vi "ShoulderExecute.vi"(8 "error in (no error)":errorcluster) -> (0 "error out":errorcluster)   [LabVIEW 2023]
doc: "Arm Execute for 2024 robot"
uses:
  <vilib>/Rock Robotics/WPI/ThirdParty/JAS_Junk/TrajLib/Trajectory_Library.lvlib
  ShoulderGetSetpointEnum.ctl
  Unused_OldRobot/ShoulderNetworkingGlobal.vi
  ShoulderGlobal.vi
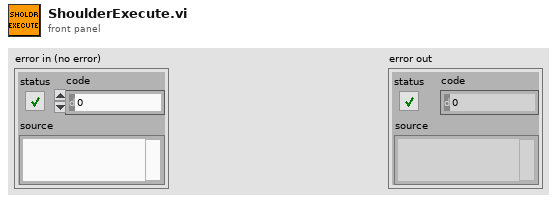
[diagram p1: front panel]
types:
  T1 = typedef "WPI_MotorControlDeviceRef.ctl" = cluster{"DeviceStatus":errorcluster, "Type":T2, "PWM":cluster{"PWM Channel":T3, "DeadBand":T4}, "CAN":cluster{"Device Number":u8, "SetOutput VI Ref":variant, "GetOutput VI Ref":variant, "Enable VI Ref":variant, "Disable VI Ref":variant, "Data":variant}, "Invert":bool, "DIO PWM":cluster{"PWM \"Enable\" Channel":T3, "DIOChannel":T5, "PWM Rate":dbl}}
  T2 = typedef "WPI_MotorControlType.ctl" = enum16{"PWM", "CAN", "DIO PWM"}
  T3 = typedef "FPGA_DIOPWMChannel.ctl" = enum8{"PWM 0", "PWM 1", "PWM 2", "PWM 3", "PWM 4", "PWM 5", "PWM 6", "PWM 7", "PWM 8", "PWM 9", "PWM MXP 0", "PWM MXP 1", "PWM MXP 2", "PWM MXP 3", "PWM MXP 4", "PWM MXP 5", "PWM MXP 6", "PWM MXP 7", "PWM MXP 8", "PWM MXP 9", "Invalid"}
  T4 = typedef "WPI_PWMDeadband.ctl" = cluster{"Name":string, "maxPositivePwm":i32, "minPositivePwm":i32, "centerPwm":i32, "maxNegativePwm":i32, "minNegativePwm":i32, "angularRange":u16}
  T5 = typedef "FPGA_DIOChannel.ctl" = enum8{"DIO 0", "DIO 1", "DIO 2", "DIO 3", "DIO 4", "DIO 5", "DIO 6", "DIO 7", "DIO 8", "DIO 9", "DIO MXP 0", "DIO MXP 1", "DIO MXP 2", "DIO MXP 3", "DIO MXP 4", "DIO MXP 5", "DIO MXP 6", "DIO MXP 7", "DIO MXP 8", "DIO MXP 9", "DIO MXP 10", "DIO MXP 11", "DIO MXP 12", "DIO MXP 13", "DIO MXP 14", "DIO MXP 15", "SPI Port CS1", "SPI Port CS2", "SPI Port CS3", "SPI Port MISO", "SPI Port MOSI", "Invalid"}
  T6 = typedef "WPI_SwitchDevRef.ctl" = cluster{"DevStatus":errorcluster, "DIO Channel":T5, "CntIndex":T7, "Normally Closed":bool}
  T7 = typedef "FPGA_CounterCtrSystemIndex.ctl" = enum8{"Ctr 0", "Ctr 1", "Ctr 2", "Ctr 3", "Ctr 4", "Ctr 5", "Ctr 6", "Ctr 7", "Invalid"}
  T8 = typedef "ShoulderGetSetpointEnum.ctl" = enum16{"ShoulderRest", "ShoulderSpeaker", "ShoulderAmp"}
  T9 = typedef "Trajectory_Library.lvlib/PosCtrl_Tuning_Type.ctl" = cluster{"Slope":dbl, "Offset":dbl, "Error Deadband":dbl, "At Reference Count":i32, "Negate Output":bool, "Max Allowd Position":dbl, "Min Allowd Position":dbl}
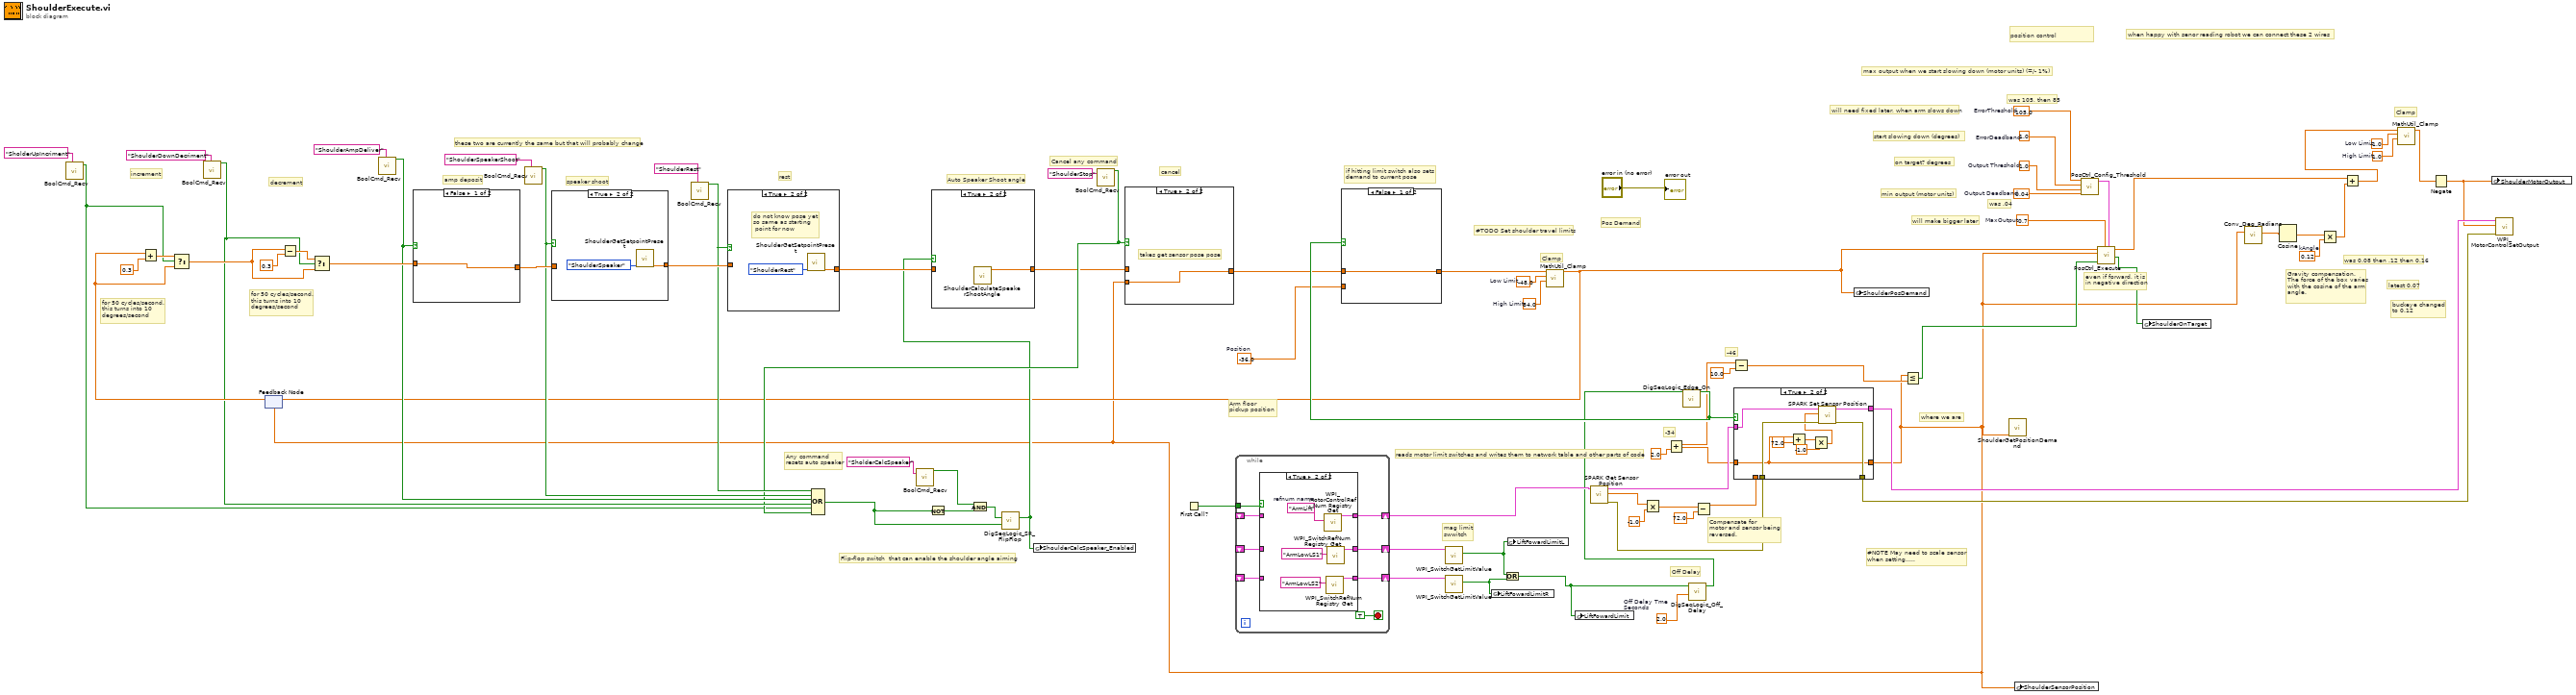
[diagram p0: block diagram]
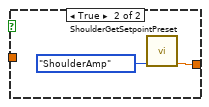
[diagram p8: hidden frame]
diagram:
  w28 = 84.0  # High Limit
  w33 = 2.0  # Off Delay Tme Seconds
  w43 = 1.0  # High Limit
  w42 = -1.0  # Low Limit
  w36 = -36.0  # Position
  w61 = 0.12  # kAngle
  w72 = -48.0  # Low Limit
  w79 = 0.7  # MaxOutput
  w77 = 105.0  # ErrorThreshold
  w76 = 1.0  # ErrorDeadband
  w75 = 1.0  # Output Threshold
  w74 = 0.04  # Output Deadband
  # "#TODO Set shoulder travel limits"
  # "Auto Speaker Shoot angle"
  # "Any command\nresets auto speaker"
  # "for 50 cycles/second.\nthis turns into 10 \ndegrees/second"
  # "for 50 cycles/second.\nthis turns into 10 \ndegrees/second"
  # "increment"
  # "buckeye changed\nto 0.12"
  # "latest 0.07"
  # "Flip-flop switch  that can enable the shoulder angle aiming"
  # "#NOTE May need to scale sensor \nwhen setting....."
  # "Off Delay"
  # "mag limit\nswwitch"
  # "-34"
  # "-46"
  # "Pos Demand"
  # "Clamp"
  # "was 105, then 85"
  # "was .04"
  # "was 0.08 then .12 then 0.16"
  # "Arm floor\npickup position"
  # "Gravity compensation.\nThe force of the box varies\nwith the cosine of the arm\nangle."
  # "Compensate for\nmotor and sensor being\nreversed."
  # "even if forward, it is \nin negative direction"
  # "if hitting limit switch also sets \ndemand to current pose"
  # "these two are currently the same but that will probably change"
  # "Cancel any command"
  # "cancel"
  # "rest"
  # "speaker shoot"
  # "Clamp"
  # "amp deposit"
  # "decrement"
  # "when happy with senor reading robot we can connect these 2 wires"
  # "min output (motor units)"
  # "max output when we start slowing down (motor units) (=/- 1%)"
  # "on target? degrees"
  # "start slowing down (degrees)"
  # "will make bigger later"
  # "where we are"
  # "position control"
  # "will need fixed later, when arm slows down"
  # "reads motor limit switches and writes them to network table and other parts of code"
  n1 = call <vilib>:"BoolCmd_Recv.vi"("Command Name"="SholderUpIncriment") -> ("New Request"=w9:bool)  [unwired: 9 in, 1 out]
  n2 = call <vilib>:"BoolCmd_Recv.vi"("Command Name"="ShoulderDownDecriment") -> ("New Request"=w11:bool)  [unwired: 9 in, 1 out]
  n3 = call <vilib>:"BoolCmd_Recv.vi"("Command Name"="ShoulderAmpDeliver") -> ("New Request"=w12:bool)  [unwired: 9 in, 1 out]
  n4 = call <vilib>:"BoolCmd_Recv.vi"("Command Name"="ShoulderSpeakerShoot") -> ("New Request"=w13:bool)  [unwired: 9 in, 1 out]
  n5 = call <vilib>:"BoolCmd_Recv.vi"("Command Name"="ShoulderRest") -> ("New Request"=w14:bool)  [unwired: 9 in, 1 out]
  n6 = call <vilib>:"BoolCmd_Recv.vi"("Command Name"="SholderCalcSpeaker") -> ("New Request"=w15:bool)  [unwired: 9 in, 1 out]
  n7 = call <vilib>:"BoolCmd_Recv.vi"("Command Name"="ShoulderStop") -> ("New Request"=w10:bool)  [unwired: 9 in, 1 out]
  n8 = Compound Arithmetic op=OR(w14, w13, w12, w11, w9, w10) -> (w8:bool)
  n9 = Not(x=w8) -> (.not. x?=w30:bool)
  n10 = And(x=w15, y=w30) -> (x .and. y?=w29:bool)
  n11 = call <vilib>:"DigSeqLogic_SR_FlipFlop.vi"("Set"=w29, "Reset"=w8) -> ("Output"=w6:bool)  [unwired: 12 in, 1 out]
  n12 = global write "ShoulderGlobal.vi" "ShoulderCalcSpeaker_Enabled"(w6) -> ()
  n13 = First Call?() -> (First Call?: T/F=w49:bool)
  n14 = while {
    tunnel: w49 -> [w86]
    shift-right: [w87] -> w44
    shift-left: _ -> [w84]
    shift-right: [w83] -> w47
    shift-left: _ -> [w82]
    shift-right: [w81] -> w27
    shift-left: _ -> [w80]
    stop <- TRUE stop-if-true
    n15 = case shown="True" w86 {
      tunnel: [w90 w96] -> w87
      tunnel: w84 -> [w90 _]
      tunnel: [w89 w93] -> w83
      tunnel: w82 -> [w89 _]
      tunnel: [w88 w91] -> w81
      tunnel: w80 -> [w88 _]
      frame False {
      }
      frame True {
        w95 = "ArmLift"  # refnum name
        n16 = call <vilib>:"WPI_MotorControlRefNum Registry Get.vi"("refnum name"=w95) -> ("MotorControlDevRef"=w96:T1)  [unwired: 9 in, 1 out]
        n17 = call <vilib>:"WPI_SwitchRefNum Registry Get.vi"("refnum name"="ArmLowLS2") -> ("SwitchDevRef"=w91:T6)  [unwired: 9 in, 1 out]
        n18 = call <vilib>:"WPI_SwitchRefNum Registry Get.vi"("refnum name"="ArmLowLS1") -> ("SwitchDevRef"=w93:T6)  [unwired: 9 in, 1 out]
      }
    }
  }
  n19 = call <vilib>:"WPI_SwitchGetLimitValue.vi"("SwitchDevRef"=w47) -> ("Switch Pressed"=w26:bool)  [unwired: 8 in, 2 out]
  n20 = call <vilib>:"WPI_SwitchGetLimitValue.vi"("SwitchDevRef"=w27) -> ("Switch Pressed"=w25:bool)  [unwired: 8 in, 2 out]
  n21 = global write "ShoulderNetworkingGlobal.vi" "LiftFowardLimitR"(w25) -> ()
  n22 = Or(x=w26, y=w25) -> (x .or. y?=w24:bool)
  n23 = global write "ShoulderNetworkingGlobal.vi" "LiftFowardLimitL"(w26) -> ()
  n24 = global write "ShoulderNetworkingGlobal.vi" "LiftFowardLimit"(w24) -> ()
  n25 = call <vilib>:"SPARK Get Sensor Position.vi"("MotorControlDevRef in"=w44) -> ("error out"=w48:errorcluster, "Sensor Position"=w57:dbl, "MotorControlDevRef out"=w58:T1)  [unwired: 7 in, 1 out]
  n26 = Multiply(x=w57, y=-1.0) -> (x*y=w55:dbl)
  n27 = Add(y=2.0) -> (x=w1:dbl, x+y=w39:dbl)
  n28 = call <vilib>:"DigSeqLogic_Off_Delay.vi"("Delay"=w33, "Input"=w24) -> ("Output"=w32:bool)  [unwired: 8 in, 1 out]
  n29 = call <vilib>:"DigSeqLogic_Edge_On.vi"("Input"=w32) -> ("On Edge"=w52:bool)  [unwired: 10 in]
  n30 = Subtract(x=w55, y=72.0) -> (x-y=w53:dbl)
  n31 = Subtract(x=w1, y=10.0) -> (x-y=w34:dbl)
  n32 = call "ShoulderGetPositionDemand.vi"() -> ("ShoulderPosDmd"=w2:dbl)  [unwired: 11 in]
  n33 = feedback #1(w2) -> (w73:dbl)
  n34 = Add(x=w73, y=0.3) -> (x+y=w20:dbl)
  n35 = Select(t=w20, s=w9, f=w73) -> (s? t:f=w19:dbl)
  n36 = Subtract(x=w19, y=0.3) -> (x-y=w17:dbl)
  n37 = Select(t=w17, s=w11, f=w19) -> (s? t:f=w23:dbl)
  n38 = case shown="False" w12 {
    tunnel: w23 -> [w97 _]
    tunnel: [w97 w98] -> w71
    frame False {
    }
    frame True {
      n39 = call "ShoulderGetSetpointPreset.vi"("SholdrSetpoints"=ShoulderGetSetpointEnum."ShoulderAmp" ("ArmSetpoints")) -> ("Setpoint"=w98:dbl)  [unwired: 10 in]
    }
  }
  n40 = case shown="True" w13 {
    tunnel: w71 -> [w100 _]
    tunnel: [w100 w102] -> w22
    frame False {
    }
    frame True {
      n41 = call "ShoulderGetSetpointPreset.vi"("SholdrSetpoints"=ShoulderGetSetpointEnum."ShoulderSpeaker") -> ("Setpoint"=w102:dbl)  [unwired: 10 in]
    }
  }
  n42 = case shown="True" w14 {
    tunnel: w22 -> [w103 _]
    tunnel: [w103 w105] -> w16
    frame False {
    }
    frame True {
      # "do not know pose yet \nso same as starting\n point for now"
      n43 = call "ShoulderGetSetpointPreset.vi"("SholdrSetpoints"=ShoulderGetSetpointEnum."ShoulderRest") -> ("Setpoint"=w105:dbl)  [unwired: 10 in]
    }
  }
  n44 = case shown="True" w6 {
    tunnel: w16 -> [w106 _]
    tunnel: [w106 w107] -> w7
    frame False {
    }
    frame True {
      n45 = call "ShoulderCalculateSpeakerShootAngle.vi"() -> ("ShoulderDesiredAngle (degrees)"=w107:dbl)  [unwired: 11 in]
    }
  }
  n46 = case shown="True" w10 {
    tunnel: w7 -> [w108 _]
    tunnel: [w108 w109] -> w50
    tunnel: w2 -> [_ w109]
    frame False {
    }
    frame True {
      # "takes get sensor pose pose"
    }
  }
  n47 = case shown="False" w52 {
    tunnel: w36 -> [_ w111]
    tunnel: [w110 w111] -> w51
    tunnel: w50 -> [w110 _]
    frame False {
    }
    frame True {
    }
  }
  n48 = call <vilib>:"MathUtil_Clamp.vi"("High Limit"=w28, "Low Limit"=w72, "Value"=w51) -> ("Result"=w5:dbl)  [unwired: 8 in]
  n49 = feedback-in #1(w5) -> ()
  n50 = case shown="True" w52 {
    tunnel: [w113 w123] -> w46
    tunnel: w2 -> [w114 w119]
    tunnel: w53 -> [w114 _]
    tunnel: w58 -> [w113 w122]
    tunnel: w39 -> [_ w119]
    tunnel: w48 -> [w112 w121]
    tunnel: [w112 w120] -> w45
    frame False {
    }
    frame True {
      n51 = Add(x=w119, y=72.0) -> (x+y=w118:dbl)
      n52 = Multiply(x=w118, y=-1.0) -> (x*y=w115:dbl)
      n53 = call <vilib>:"SPARK Set Sensor Position.vi"("error in"=w121, "Position"=w115, "MotorControlDeviceRef"=w122) -> ("error out"=w120:errorcluster, "MotorControlDeviceRef"=w123:T1)  [unwired: 7 in]
    }
  }
  n54 = global write "ShoulderGlobal.vi" "ShoulderPosDemand"(w5) -> ()
  n55 = Less Or Equal?(x=w2, y=w34) -> (x <= y?=w37:bool)
  n56 = global write "ShoulderGlobal.vi" "ShoulderSensorPosition"(w2) -> ()
  n57 = call <vilib>:"PosCtrl_Config_Threshold.vi"("Output Deadband"=w74, "Output Threshold"=w75, "ErrorDeadband"=w76, "ErrorThreshold"=w77) -> ("PosCtrl_Config_Params"=w78:T9)  [unwired: 7 in]
  n58 = call <vilib>:"PosCtrl_Execute.vi"("PosCtrl_Config_Params"=w78, "MaxOutput"=w79, "Rev Limit Switch"=w37, "CurrentPosition"=w2, "TargetPosition"=w5) -> ("OnTarget"=w4:bool, "Output"=w63:dbl)  [unwired: 4 in, 1 out]
  n59 = global write "ShoulderGlobal.vi" "ShoulderOnTarget"(w4) -> ()
  n60 = call <vilib>:"Conv_Deg_Radians.vi"("Degress"=w2) -> ("Radians"=w59:dbl)  [unwired: 10 in]
  n61 = Cosine(x=w59) -> (cos(x)=w60:dbl)
  n62 = Multiply(x=w60, y=w61) -> (x*y=w62:dbl)
  n63 = Add(x=w63, y=w62) -> (x+y=w41:dbl)
  n64 = call <vilib>:"MathUtil_Clamp.vi"("High Limit"=w43, "Low Limit"=w42, "Value"=w41) -> ("Result"=w40:dbl)  [unwired: 8 in]
  n65 = Negate(x=w40) -> (-x=w3:dbl)
  n66 = global write "ShoulderGlobal.vi" "ShoulderMotorOutput"(w3) -> ()
  n67 = call <vilib>:"WPI_MotorControlSetOutput.vi"("error in (no error)"=w45, "Output"=w3, "MotorControlDevRef"=w46) -> ()  [unwired: 6 in, 3 out]
  "error out" <- "error in (no error)"
